vi "6812B_AC_pwrcur.vi"() -> ()   [LabVIEW 2019]
doc: "Shows how to generate a standard output."
uses:
  <instrlib>/Agilent 681x Series/Public/Data/Read Single Measurement (Current).vi
  <instrlib>/Agilent 681x Series/Public/Data/Low Level/Fetch Single Measurement (Power).vi
  <instrlib>/Agilent 681x Series/Agilent 681x Series.lvlib
panel:
  in  "STOP":bool
  out "Total Power":dbl
  out "Power Factor":dbl
  out "Reactive Power":dbl
  out "Apparent Power":dbl
  out "Real Power":dbl
  out "DC Power":dbl
  out "enmed":bool
  out "Name":string
  in  "Sense Source (0: Internal)":u16(ring) items=["Internal", "External"]
  in  "Sample Spacing (25 us)":dbl=2.5e-05 format="%^.2g"
  in  "Relative Trigger Samples (0)":i32
  out "Peak Current":dbl
  out "AC + DC RMS Current":dbl
  out "AC RMS Current":dbl
  out "DC Current":dbl
  in  "Pulse Characteristic Value (%)":dbl=50.0 format="%#.4g"
  in  "Pulse Characteristic (0: Duty Cycle)":u16(ring) items=["Duty Cycle", "Pulse Width"]
  in  "Period (s)":dbl=0.03333 format="%#.4g"
  in  "Trigger Delay (s)":dbl format="%#.5g"
  in  "Pulse Count":dbl=1.0 format="%#.4g"
  in  "Voltage Mode (0: Fix)":u16(ring) items=["Fixed", "Step", "Pulse", "List"]
  in  "Triggered Voltage Amplitude (V)":dbl=1.0 format="%#.4g"
  in  "Peak Current Limit (13 A)":dbl=13.0 format="%#.4g"
  in  "RMS Current Limit (1 A)":dbl=1.0 format="%#.4g"
  in  "Voltage Amplitude (1.0 V)":dbl=1.0 format="%#.4g"
  in  "Output Frequency (60 Hz)":dbl=60.0 format="%#.4g"
  in  "Output Waveform Type (0: Sinusoid)":u16(ring) items=["Sinusoid", "Square", "Clipped Sinusoid", "User Specified"]
  in  "Serial Configuration":T1={"Baud Rate"=9600, "Parity"=0, "Data Bits"=8} {"Data Bits" items=["7"=7, "8"=8]; "Parity" items=["None", "Odd", "Even", "Mark", "Space"]; "Baud Rate" items=["300"=300, "600"=600, "1200"=1200, "2400"=2400, "4800"=4800, "9600"=9600]}
  in  "VISA resource name":refnum<visa-resource-name>
  # "(c) 2008-2021 National Instruments Corp.  ALL RIGHTS RESERVED."
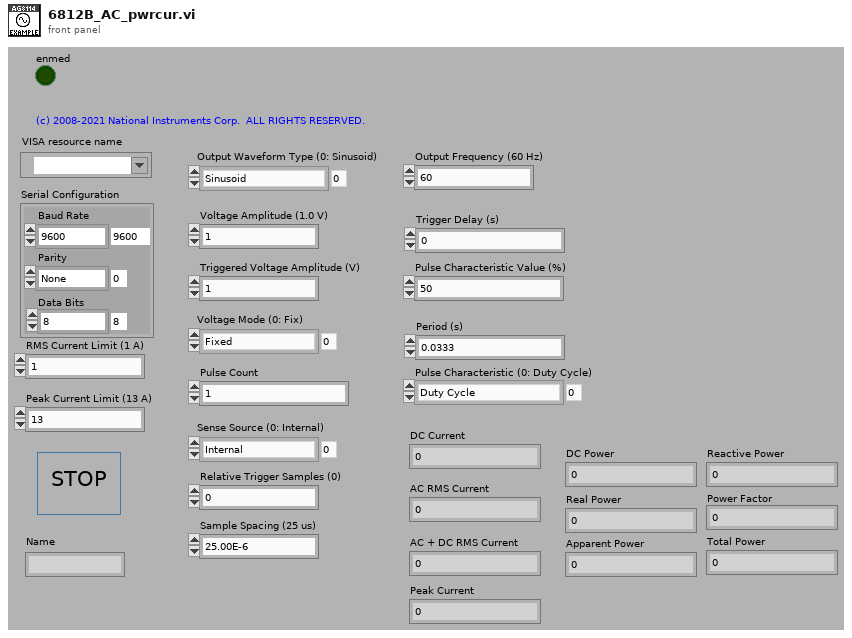
[diagram p1: front panel]
types:
  T1 = cluster{"Baud Rate":u32, "Parity":u16, "Data Bits":u16}
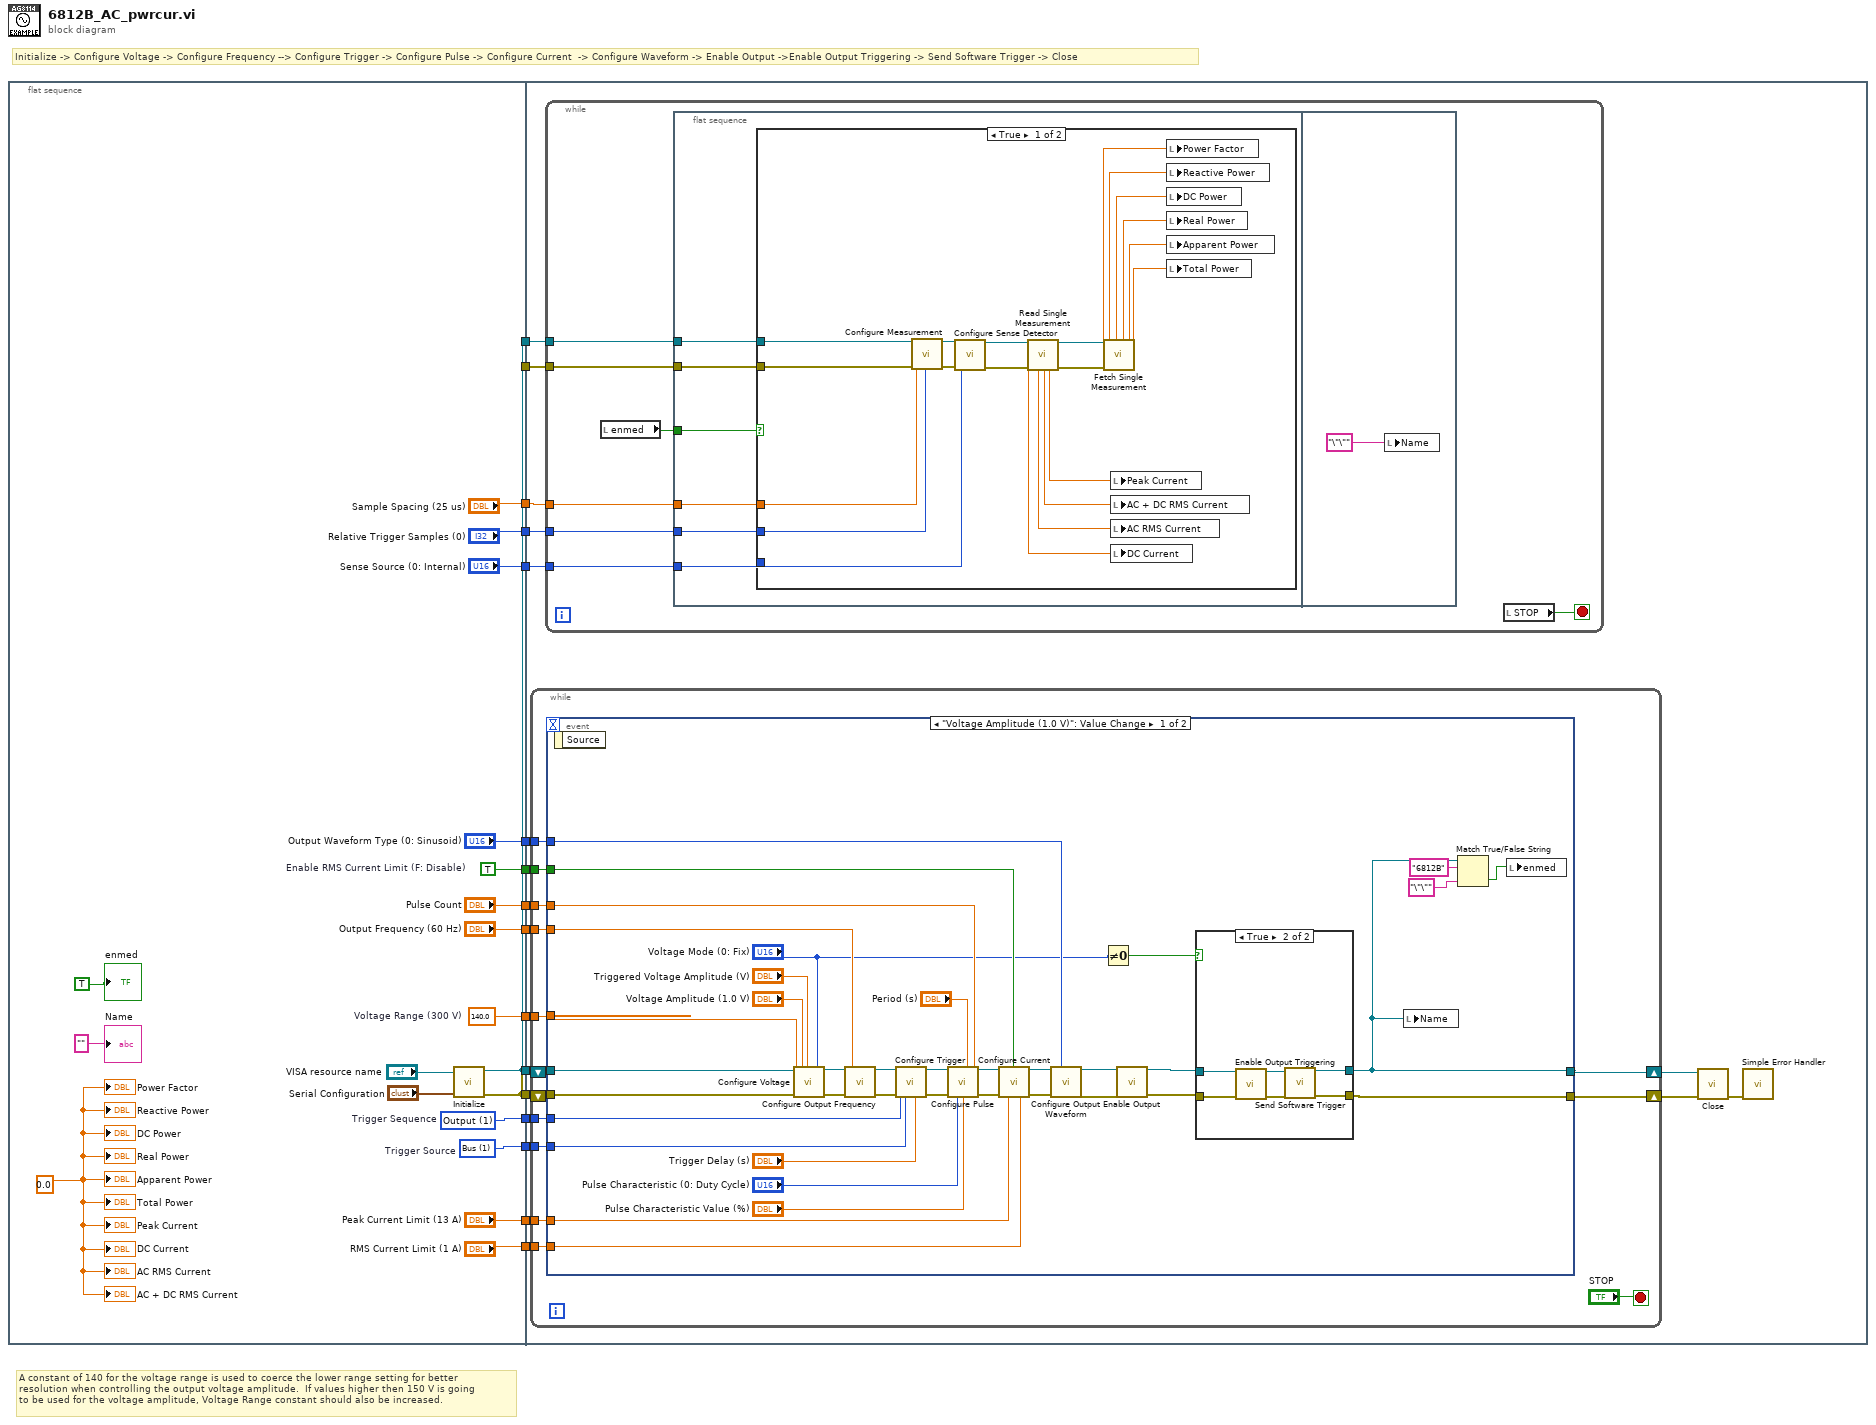
[diagram p0: block diagram]
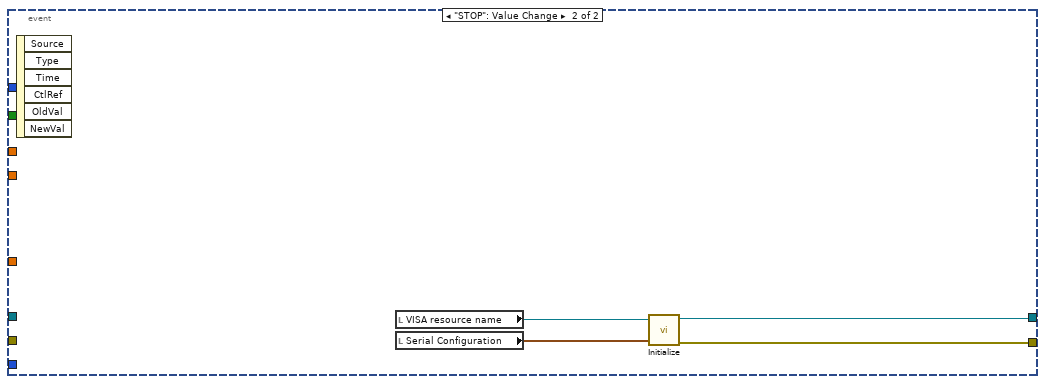
[diagram p4: hidden frame]
diagram:
  # "Initialize -> Configure Voltage -> Configure Frequency --> Configure Trigger -> Configure Pulse -> Configure Current  -> Configure Waveform -> Enable Output ->Enable Output Triggering -> Send Software Trigger -> Close"
  # "A constant of 140 for the voltage range is used to coerce the lower range setting for better\nresolution when controlling the output voltage amplitude.  If values higher then 150 V is going\nto be used for the voltage amplitude, Voltage Range constant should also be increased."
  n1 = flat-sequence {
    tunnel: [w18] -> w16
    tunnel: [w17] -> w15
    tunnel: ["Output Waveform Type (0: Sinusoid)"] -> w14
    tunnel: [w34] -> w13
    tunnel: [w33] -> w12
    tunnel: ["Output Frequency (60 Hz)"] -> w11
    tunnel: ["RMS Current Limit (1 A)"] -> w10
    tunnel: ["Peak Current Limit (13 A)"] -> w9
    tunnel: ["Pulse Count"] -> w8
    tunnel: [w26] -> w7
    tunnel: [w25] -> w6
    tunnel: ["Sense Source (0: Internal)"] -> w5
    tunnel: ["Sample Spacing (25 us)"] -> w4
    tunnel: ["Relative Trigger Samples (0)"] -> w3
    tunnel: [w18] -> w2
    tunnel: [w17] -> w1
    tunnel: w16 -> [w51]
    tunnel: w15 -> [w41]
    tunnel: w14 -> [w50]
    tunnel: w13 -> [w49]
    tunnel: w12 -> [w48]
    tunnel: w11 -> [w47]
    tunnel: w10 -> [w46]
    tunnel: w9 -> [w45]
    tunnel: w8 -> [w44]
    tunnel: w7 -> [w43]
    tunnel: w6 -> [w42]
    tunnel: w5 -> [w38]
    tunnel: w4 -> [w40]
    tunnel: w3 -> [w39]
    tunnel: w2 -> [w37]
    tunnel: w1 -> [w36]
    frame #0 {
      w19 = 0.0 ("Peak Current")
      w25 = 1 items=["Immediate", "Bus", "External", "Phase", "Trigger Out"]  # Trigger Source
      w26 = 1 items=["Output"=1, "Synchronous Source"=2, "Measurement"=3]  # Trigger Sequence
      w33 = TRUE  # Enable RMS Current Limit (F: Disable)
      w34 = 140.0  # Voltage Range (300 V)
      n2 = call <instrlib>:"Initialize.vi"("Serial Configuration"="Serial Configuration", "VISA resource name"="VISA resource name") -> ("error out"=w17:errorcluster, "VISA resource name out"=w18:refnum<visa-resource-name>)  [unwired: 8 in]
      "DC Current" <- w19
      "AC RMS Current" <- w19
      "AC + DC RMS Current" <- w19
      "Peak Current" <- w19
      "Name" <- "" ("Meas")
      "enmed" <- TRUE ("med")
      "DC Power" <- w19
      "Real Power" <- w19
      "Apparent Power" <- w19
      "Reactive Power" <- w19
      "Power Factor" <- w19
      "Total Power" <- w19
    }
    frame #1 {
      n3 = while {
        tunnel: w50 -> [w99]
        tunnel: w49 -> [w98]
        tunnel: w48 -> [w97]
        tunnel: w47 -> [w96]
        tunnel: w46 -> [w95]
        tunnel: w45 -> [w94]
        shift-right: [w103] -> w53
        shift-left: w51 -> [w101]
        shift-right: [w102] -> w52
        shift-left: w41 -> [w100]
        tunnel: w44 -> [w93]
        tunnel: w43 -> [w92]
        tunnel: w42 -> [w91]
        stop <- "STOP" stop-if-true
        n4 = event shown="[0] \"Voltage Amplitude (1.0 V)\": Value Change" {
          selector: _ -> [_ _]
          dyn-events: _ -> [_ _]
          timeout: _ -> [_ _]
          tunnel: w101 -> [w117 _]
          tunnel: w100 -> [w116 _]
          tunnel: w99 -> [w141 _]
          tunnel: w98 -> [w140 _]
          tunnel: w97 -> [w139 _]
          tunnel: [w111 w153] -> w102
          tunnel: [w107 w152] -> w103
          tunnel: w96 -> [w133 _]
          tunnel: w95 -> [w138 _]
          tunnel: w94 -> [w137 _]
          tunnel: w93 -> [w124 _]
          tunnel: w92 -> [w120 _]
          tunnel: w91 -> [w114 _]
          event "Voltage Amplitude (1.0 V)": Value Change {
            n5 = event-data() -> ()  [unwired: 1 in, 1 out]
            n6 = call <instrlib>:"Configure Voltage.vi"("VISA resource name"=w117, "Triggered Voltage Amplitude (1.0 V)"="Triggered Voltage Amplitude (V)", "Voltage Range (300 V)"=w140, "Voltage Amplitude (1.0 V)"="Voltage Amplitude (1.0 V)", "Voltage Mode (0: Fix)"="Voltage Mode (0: Fix)", "error in (no error)"=w116) -> ("VISA resource name out"=w135:refnum<visa-resource-name>, "error out"=w134:errorcluster)  [unwired: 8 in]
            n7 = call <instrlib>:"Configure Output Frequency.vi"("VISA resource name"=w135, "Output Frequency (60 Hz)"=w133, "error in (no error)"=w134) -> ("VISA resource name out"=w132:refnum<visa-resource-name>, "error out"=w131:errorcluster)  [unwired: 11 in]
            n8 = call <instrlib>:"Configure Trigger.vi"("VISA resource name"=w132, "Trigger Sequence (1: Output 1)"=w120, "Trigger Source (0: Immediate)"=w114, "error in (no error)"=w131, "Trigger Delay (0 s)"="Trigger Delay (s)") -> ("VISA resource name out"=w130:refnum<visa-resource-name>, "error out"=w129:errorcluster)  [unwired: 9 in]
            n9 = call <instrlib>:"Configure Pulse.vi"("VISA resource name"=w130, "Pulse Count (1)"=w124, "Period (0.0333 s)"="Period (s)", "error in (no error)"=w129, "Pulse Characteristic (0: Duty Cycle)"="Pulse Characteristic (0: Duty Cycle)", "Pulse Characteristic Value (50)"="Pulse Characteristic Value (%)") -> ("VISA resource name out"=w128:refnum<visa-resource-name>, "error out"=w127:errorcluster)  [unwired: 8 in]
            n10 = call <instrlib>:"Configure Current.vi"("VISA resource name"=w128, "Enable RMS Current Limit (F: Disable)"=w139, "RMS Current Limit (1 A)"=w138, "error in (no error)"=w127, "Peak Current Limit (13 A)"=w137) -> ("VISA resource name out"=w126:refnum<visa-resource-name>, "error out"=w125:errorcluster)  [unwired: 9 in]
            n11 = call <instrlib>:"Configure Output Waveform.vi"("VISA resource name"=w126, "Output Waveform Type (0: Sinusoid)"=w141, "error in (no error)"=w125) -> ("VISA resource name out"=w112:refnum<visa-resource-name>, "error out"=w113:errorcluster)  [unwired: 11 in]
            n12 = Not Equal To 0?(x="Voltage Mode (0: Fix)") -> (x != 0?=w109:bool)
            n13 = call <instrlib>:"Enable Output.vi"("VISA resource name"=w112, "error in (no error)"=w113) -> ("VISA resource name out"=w108:refnum<visa-resource-name>, "error out"=w110:errorcluster)  [unwired: 12 in]
            n14 = case shown="True" w109 {
              tunnel: w108 -> [w143 w148]
              tunnel: w110 -> [w142 w147]
              tunnel: [w143 w145] -> w107
              tunnel: [w142 w144] -> w111
              frame False {
              }
              frame True {
                n15 = call <instrlib>:"Enable Output Triggering.vi"("VISA resource name"=w148, "error in (no error)"=w147) -> ("VISA resource name out"=w149:refnum<visa-resource-name>, "error out"=w146:errorcluster)  [unwired: 12 in]
                n16 = call <instrlib>:"Send Software Trigger.vi"("VISA resource name"=w149, "error in (no error)"=w146) -> ("VISA resource name out"=w145:refnum<visa-resource-name>, "error out"=w144:errorcluster)  [unwired: 12 in]
              }
            }
            n17 = local write "Name"(w107) -> ()
            n18 = Match True/False String(2:"\"\"" ("false string"), 3:"6812B" ("true string"), 4:w107) -> (0:w105:bool)  [unwired: 1 out]
            n19 = local write "enmed"(w105) -> ()
          }
          event "STOP": Value Change {
            n20 = event-data() -> ()  [unwired: 1 in, 6 out]
            n21 = local read "VISA resource name"() -> (w151:refnum<visa-resource-name>)
            n22 = local read "Serial Configuration"() -> (w150:T1)
            n23 = call <instrlib>:"Initialize.vi"("Serial Configuration"=w150, "VISA resource name"=w151) -> ("error out"=w153:errorcluster, "VISA resource name out"=w152:refnum<visa-resource-name>)  [unwired: 8 in]
          }
        }
      }
      n24 = while {
        tunnel: w40 -> [w61]
        tunnel: w39 -> [w60]
        tunnel: w38 -> [w59]
        tunnel: w37 -> [w56]
        tunnel: w36 -> [w55]
        stop <- w58 stop-if-true
        n25 = local read "enmed"() -> (w57:bool)
        n26 = flat-sequence {
          tunnel: w61 -> [w67]
          tunnel: w60 -> [w66]
          tunnel: w59 -> [w65]
          tunnel: w57 -> [w64]
          tunnel: w56 -> [w63]
          tunnel: w55 -> [w62]
          frame #0 {
            n27 = case shown="True" w64 {
              tunnel: w67 -> [w88 _]
              tunnel: w66 -> [w87 _]
              tunnel: w65 -> [w86 _]
              tunnel: w63 -> [w70 _]
              tunnel: w62 -> [w69 _]
              frame True {
                n28 = call <instrlib>:"Configure Measurement.vi"("VISA resource name"=w70, "Relative Trigger Samples (0)"=w87, "Sample Spacing (25 us)"=w88, "error in (no error)"=w69) -> ("VISA resource name out"=w84:refnum<visa-resource-name>, "error out"=w85:errorcluster)  [unwired: 10 in]
                n29 = call <instrlib>:"Configure Sense Detector.vi"("VISA resource name"=w84, "Sense Source (0: Internal)"=w86, "error in (no error)"=w85) -> ("VISA resource name out"=w82:refnum<visa-resource-name>, "error out"=w83:errorcluster)  [unwired: 11 in]
                n30 = call-poly <instrlib>:"Read Single Measurement.vi"("VISA resource name"=w82, "error in (no error)"=w83) -> ("Peak Current"=w81:dbl, "VISA resource name out"=w78:refnum<visa-resource-name>, "DC Current"=w80:dbl, "AC RMS Current"=w68:dbl, "AC + DC RMS Current"=w79:dbl, "error out"=w77:errorcluster)  [unwired: 8 in]
                n31 = call-poly <instrlib>:"Fetch Single Measurement.vi"("VISA resource name"=w78, "error in (no error)"=w77) -> ("Power Factor"=w76:dbl, "Reactive Power"=w75:dbl, "DC Power"=w74:dbl, "Real Power"=w73:dbl, "Apparent Power"=w72:dbl, "Total Power"=w71:dbl)  [unwired: 6 in, 2 out]
                n32 = local write "Peak Current"(w81) -> ()
                n33 = local write "AC + DC RMS Current"(w80) -> ()
                n34 = local write "AC RMS Current"(w68) -> ()
                n35 = local write "DC Current"(w79) -> ()
                n36 = local write "Power Factor"(w76) -> ()
                n37 = local write "Reactive Power"(w75) -> ()
                n38 = local write "DC Power"(w74) -> ()
                n39 = local write "Real Power"(w73) -> ()
                n40 = local write "Apparent Power"(w72) -> ()
                n41 = local write "Total Power"(w71) -> ()
              }
              frame False {
              }
            }
          }
          frame #1 {
            n42 = local write "Name"("\"\"" ("Meas")) -> ()
          }
        }
        n43 = local read "STOP"() -> (w58:bool)
      }
      n44 = call <instrlib>:"Close.vi"("error in (no error)"=w52, "VISA resource name"=w53) -> ("error out"=w54:errorcluster)  [unwired: 9 in]
      n45 = call <vilib>:"Simple Error Handler.vi"("error in (no error)"=w54) -> ()  [unwired: 4 in, 5 out]
    }
  }
